vi "RequestFIFO3.vi"   [LabVIEW 2018]
uses:
  <vilib>/rvi/Emulation/niFpgaGetClockAttributes.vi
  <vilib>/rvi/Emulation/niFpgaSctlEmulationGetInTimedLoop.vi
  <vilib>/rvi/Emulation/niFpgaEmulationReportErrorSimple.vi
  <vilib>/rvi/interface/RandomDataEmulation/niFpgaRandomDataHandleErrors.vi
  <vilib>/rvi/Emulation/niFpgaEmulationIsFPGAContextNoSignature.vi
  <vilib>/rvi/errors/niFpgaSetErrorForExecOnDevCompSimple.vi
  <vilib>/rvi/eio/common/nirviEmuReportErrorAndStop.vi
  <vilib>/rvi/DataTransferAndStorage/Container/Common/niFpgaContainerGetUniqueNameForEmu.vi
  <vilib>/rvi/FIFO/Fifo_Resource/nirvififoEmulationSetSize.vi
  <vilib>/rvi/FIFO/Fifo_Resource/nirviFifoEmulationQueueMgr.vi
  <instcachedir>/0/nirviFifoEmulationQueueMgr_E5CAEC123FF24DC58D834DCA3CDAA9B5.lvgen/nirviFifoEmulationQueueMgr_E5CAEC123FF24DC58D834DCA3CDAA9B5_023.vi
  <vilib>/Utility/error.llb/Clear Errors.vi
  <vilib>/rvi/FIFO/Fifo_Resource/nirvififoEmulationCreateLock.vi
  <vilib>/rvi/Emulation/niFpgaProcessEmulError.vi
  <vilib>/rvi/FIFO/Fifo_Resource/nirvififoEmulationObtainLock.vi
  <vilib>/rvi/FIFO/Fifo_Resource/nirvififoEmulationReleaseLock.vi
  <vilib>/rvi/occurrence/nirviWaitOnOccurrenceBase.vi
  <vilib>/rvi/errors/nirviReportUnexpectedCaseInternalError.vi
  <vilib>/rvi/errors/nirviReportUnexpectedCaseInternalError (U32).vi
  <instcachedir>/0/nirviFifoEmulationQueueMgr_E5CAEC123FF24DC58D834DCA3CDAA9B5.lvgen/nirviFifoEmulationQueueMgr_E5CAEC123FF24DC58D834DCA3CDAA9B5_017.vi
  <vilib>/rvi/Emulation/niFpgaCriticalErrorInLSC.vi
  <vilib>/rvi/DataTransferAndStorage/Container/XNode/niFpgaContainer.xnode
  <vilib>/rvi/interface/RandomDataEmulation/nirviRandomDataFpgaReadWriteTemplate.vi
  <vilib>/rvi/FIFO/Fifo_Resource/nirvififoEmulationRead.vi
types:
  T1 = typedef "Addresses.ctl" = enum8{"NA", "Accelerometer1X", "Accelerometer1Y", "Accelerometer1Z", "Accelerometer2X", "Accelerometer2Y", "Accelerometer2Z", "Accelerometer3X", "Accelerometer3Y", "Accelerometer3Z", "Accelerometer4X", "Accelerometer4Y", "Accelerometer4Z", "Accelerometer5X", "Accelerometer5Y", "Accelerometer5Z", "Accelerometer6X", "Accelerometer6Y", "Accelerometer6Z", "Sync1", "Sync2", "Sync3", "Sync4", "Accelerometer1", "Accelerometer2", "Accelerometer3", "Accelerometer4", "Accelerometer5", "Accelerometer6", "Accelerometers", "Timestamp", "SamplePeriod"}
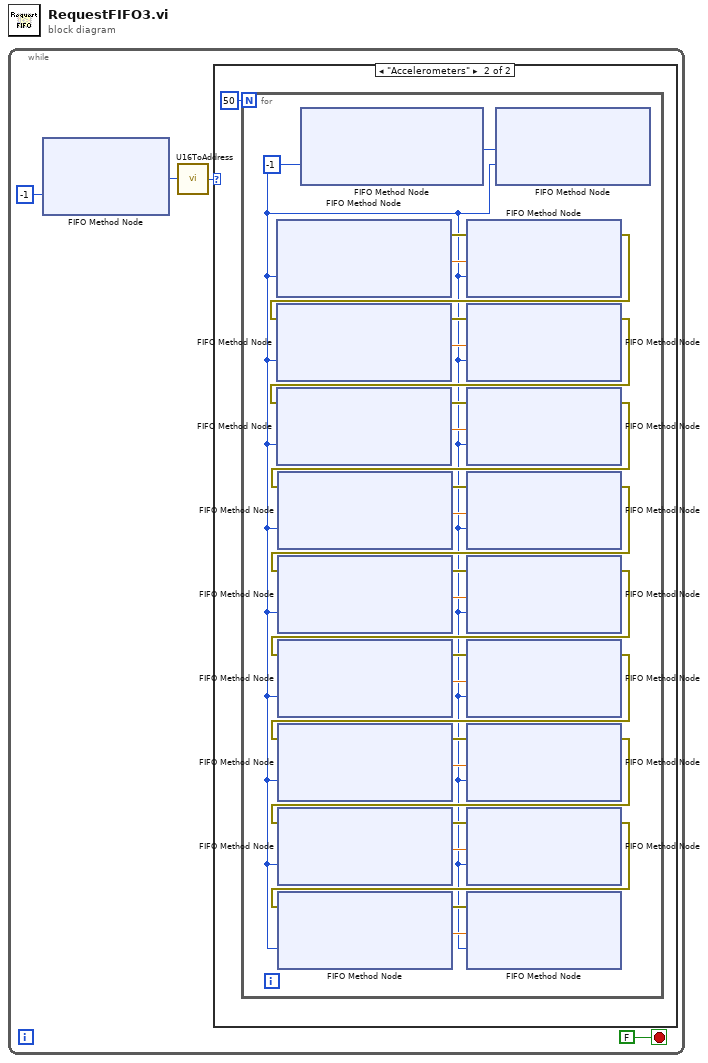
[diagram p0: block diagram]
diagram:
  n1 = while {
    stop <- FALSE stop-if-true
    n2 = xnode ("FIFO Method Node")("Timeout"=-1) -> ("Element"=w2:u16)  [unwired: 1 in, 2 out]
    n3 = call "U16ToAddress.vi"("Input"=w2) -> ("Addresses"=w1:T1)
    n4 = case shown="\"Accelerometers\"" w1 {
      frame "NA", Default {
      }
      frame "Accelerometers" {
        n5 = for {
          N: 50 -> [_]
          w7 = -1 ("Timeout")
          n6 = xnode ("FIFO Method Node")("Timeout"=w7) -> ("Element"=w33:sgl, "error out"=w32:errorcluster)  [unwired: 2 in, 2 out]
          n7 = xnode ("FIFO Method Node")("Timeout"=w7) -> ("Element"=w6:u64)  [unwired: 1 in, 2 out]
          n8 = xnode ("FIFO Method Node")("Element"=w33, "Timeout"=w7, "error in (no error)"=w32) -> ("error out"=w20:errorcluster)  [unwired: 1 in, 2 out]
          n9 = xnode ("FIFO Method Node")("Timeout"=w7, "error in (no error)"=w20) -> ("Element"=w30:sgl, "error out"=w31:errorcluster)  [unwired: 1 in, 2 out]
          n10 = xnode ("FIFO Method Node")("Element"=w30, "Timeout"=w7, "error in (no error)"=w31) -> ("error out"=w21:errorcluster)  [unwired: 1 in, 2 out]
          n11 = xnode ("FIFO Method Node")("Timeout"=w7, "error in (no error)"=w21) -> ("Element"=w29:sgl, "error out"=w28:errorcluster)  [unwired: 1 in, 2 out]
          n12 = xnode ("FIFO Method Node")("Element"=w29, "Timeout"=w7, "error in (no error)"=w28) -> ("error out"=w19:errorcluster)  [unwired: 1 in, 2 out]
          n13 = xnode ("FIFO Method Node")("Timeout"=w7, "error in (no error)"=w19) -> ("Element"=w26:sgl, "error out"=w27:errorcluster)  [unwired: 1 in, 2 out]
          n14 = xnode ("FIFO Method Node")("Element"=w26, "Timeout"=w7, "error in (no error)"=w27) -> ("error out"=w12:errorcluster)  [unwired: 1 in, 2 out]
          n15 = xnode ("FIFO Method Node")("Timeout"=w7, "error in (no error)"=w12) -> ("Element"=w24:sgl, "error out"=w25:errorcluster)  [unwired: 1 in, 2 out]
          n16 = xnode ("FIFO Method Node")("Element"=w24, "Timeout"=w7, "error in (no error)"=w25) -> ("error out"=w11:errorcluster)  [unwired: 1 in, 2 out]
          n17 = xnode ("FIFO Method Node")("Timeout"=w7, "error in (no error)"=w11) -> ("Element"=w22:sgl, "error out"=w23:errorcluster)  [unwired: 1 in, 2 out]
          n18 = xnode ("FIFO Method Node")("Element"=w22, "Timeout"=w7, "error in (no error)"=w23) -> ("error out"=w10:errorcluster)  [unwired: 1 in, 2 out]
          n19 = xnode ("FIFO Method Node")("Timeout"=w7, "error in (no error)"=w10) -> ("Element"=w15:sgl, "error out"=w16:errorcluster)  [unwired: 1 in, 2 out]
          n20 = xnode ("FIFO Method Node")("Element"=w15, "Timeout"=w7, "error in (no error)"=w16) -> ("error out"=w9:errorcluster)  [unwired: 1 in, 2 out]
          n21 = xnode ("FIFO Method Node")("Timeout"=w7, "error in (no error)"=w9) -> ("Element"=w13:sgl, "error out"=w14:errorcluster)  [unwired: 1 in, 2 out]
          n22 = xnode ("FIFO Method Node")("Element"=w13, "Timeout"=w7, "error in (no error)"=w14) -> ("error out"=w8:errorcluster)  [unwired: 1 in, 2 out]
          n23 = xnode ("FIFO Method Node")("Timeout"=w7, "error in (no error)"=w8) -> ("Element"=w18:sgl, "error out"=w17:errorcluster)  [unwired: 1 in, 2 out]
          n24 = xnode ("FIFO Method Node")("Element"=w18, "Timeout"=w7, "error in (no error)"=w17) -> ()  [unwired: 1 in, 3 out]
          n25 = xnode ("FIFO Method Node")("Element"=w6, "Timeout"=w7) -> ()  [unwired: 1 in, 2 out]
        }
      }
    }
  }
